vi "main(Test DQMH modules).bak.vi"() -> ()   [LabVIEW 2018, in "Application.lvlib"] (continued)
        n2853 = To Variant(anything=bool[] [FALSE, FALSE, FALSE, FALSE, FALSE, TRUE]) -> (Variant=w6353:variant)
        n2854 = To Variant(anything=T6."demux1_10_channel2" ("demux1_10(x6)_encode")) -> (Variant=w6357:variant)
        n2855 = To Variant(anything=T4."mux6_1_channel6_3" ("mux6_1(3wires)_encode")) -> (Variant=w6361:variant)
        n2856 = To Variant(anything=T5."mux10_1_channel2" ("mux10_1(x6)_encode")) -> (Variant=w6363:variant)
        n2857 = Bundle By Name(cluster=w6356, "command"="MEAS.mux10-1", "command data"=w6363) -> (w6351:T11)
        n2858 = Bundle By Name(cluster=w6356, "command"="MEAS.mux6_1", "command data"=w6361) -> (w6350:T11)
        n2859 = Bundle By Name(cluster=w6356, "command"="MEAS.demux1-10", "command data"=w6357) -> (w6349:T11)
        n2860 = Bundle By Name(cluster=w6356, "command"="MEAS.eMIC", "command data"=w6353) -> (w6348:T11)
        n2861 = Bundle By Name(cluster=w6356, "command"="MEAS.AllRelaysOFF") -> (w6352:T11)
        n2862 = Build Array(w6352, w6351, w6350, w6349, w6348) -> (w6343:T11[])
        n2863 = Bundle By Name(cluster=w6330, "command"="MEAS.requestAC", "command data"=w6324) -> (w6344:T11)
        n2864 = Bundle By Name(cluster=w6330, "command"="Apps.WaitForEvent", "command data"=w6324) -> (w6329:T11)
        n2865 = Bundle By Name(cluster=w6330, "command"="MEAS.DMM dual read") -> (w6345:T11)
        n2866 = Bundle By Name(cluster=w6330, "command"="Apps.UI Update 1") -> (w6331:T11)
        n2867 = Build Array(w6345, w6344, w6329, w6331) -> (w6342:T11[])
        n2868 = Build Array (concatenate)(w6343, w6342) -> (w6341:T11[])
        n2869 = for {
          tunnel: w6341 -> [w6379] mode=indexing
          tunnel: w6336 -> [w6380]
          tunnel: [w6376] -> w6339 mode=indexing
          n2870 = Unbundle By Name(w6379) -> ("command"=w6378:string, "command data"=w6377:variant)
          n2871 = call "App enquece.vi"("command data"=w6377, "command"=w6378, "queue in"=w6380) -> ("error out"=w6376:errorcluster)  [unwired: 7 in, 1 out]
        }
        n2872 = Merge Errors(w6340, w6339) -> (w6338:errorcluster)
      }
      frame "Test DRV 13A" {
        w6387 = T11 {"command"="", "command data"=variant} ("element")
        w6382 = 13 ("DUT index(0-59)")
        w6413 = T11 {"command"="", "command data"=variant} ("element")
        n2873 = disable-structure shown="LOGGING==TRUE" {
          disable-tunnel: w6391 -> [w6429 _]
          frame condition #0 (active) {
            n2874 = Empty String/Path?(string/path=w6429) -> (empty?=w6432:bool)
            n2875 = Select(t="Quece timeout", s=w6432, f=w6429) -> (s? t:f=w6428:string)
            n2876 = call "string log (SubVI).vi"("Enum"=enum16{"Init", "Log", "Read"}."Log", "state Name"=w6428) -> ()  [unwired: 8 in, 2 out]
          }
          frame condition #1 {
          }
        }
        n2877 = Flush Queue(queue=w6392) -> (queue out=w6393:refnum<queue>)  [unwired: 1 in, 2 out]
        n2878 = Decrement(x=w6382) -> (x-1=w6385:i32)
        n2879 = Index Array(array=w6381, index=w6385) -> (element=w6383:refnum<vi>)
        n2880 = property class="ColBox"(reference=w6383, "Value"=u32 10000536 ("DRV 1")) -> ()  [unwired: 1 in, 2 out]
        n2881 = To Variant(anything=bool[] [TRUE, FALSE, FALSE, FALSE, FALSE, FALSE]) -> (Variant=w6410:variant)
        n2882 = To Variant(anything=T6."demux1_10_channel3" ("demux1_10(x6)_encode")) -> (Variant=w6414:variant)
        n2883 = To Variant(anything=T4."mux6_1_channel1_3" ("mux6_1(3wires)_encode")) -> (Variant=w6418:variant)
        n2884 = To Variant(anything=T5."mux10_1_channel3" ("mux10_1(x6)_encode")) -> (Variant=w6420:variant)
        n2885 = Bundle By Name(cluster=w6413, "command"="MEAS.mux10-1", "command data"=w6420) -> (w6408:T11)
        n2886 = Bundle By Name(cluster=w6413, "command"="MEAS.mux6_1", "command data"=w6418) -> (w6407:T11)
        n2887 = Bundle By Name(cluster=w6413, "command"="MEAS.demux1-10", "command data"=w6414) -> (w6406:T11)
        n2888 = Bundle By Name(cluster=w6413, "command"="MEAS.eMIC", "command data"=w6410) -> (w6405:T11)
        n2889 = Bundle By Name(cluster=w6413, "command"="MEAS.AllRelaysOFF") -> (w6409:T11)
        n2890 = Build Array(w6409, w6408, w6407, w6406, w6405) -> (w6400:T11[])
        n2891 = Bundle By Name(cluster=w6387, "command"="MEAS.requestAC", "command data"=w6382) -> (w6401:T11)
        n2892 = Bundle By Name(cluster=w6387, "command"="Apps.WaitForEvent", "command data"=w6382) -> (w6386:T11)
        n2893 = Bundle By Name(cluster=w6387, "command"="MEAS.DMM dual read") -> (w6402:T11)
        n2894 = Bundle By Name(cluster=w6387, "command"="Apps.UI Update 1") -> (w6388:T11)
        n2895 = Build Array(w6402, w6401, w6386, w6388) -> (w6399:T11[])
        n2896 = Build Array (concatenate)(w6400, w6399) -> (w6398:T11[])
        n2897 = for {
          tunnel: w6398 -> [w6436] mode=indexing
          tunnel: w6393 -> [w6437]
          tunnel: [w6433] -> w6396 mode=indexing
          n2898 = Unbundle By Name(w6436) -> ("command"=w6435:string, "command data"=w6434:variant)
          n2899 = call "App enquece.vi"("command data"=w6434, "command"=w6435, "queue in"=w6437) -> ("error out"=w6433:errorcluster)  [unwired: 7 in, 1 out]
        }
        n2900 = Merge Errors(w6397, w6396) -> (w6395:errorcluster)
      }
      frame "Test DRV 14A" {
        w6444 = T11 {"command"="", "command data"=variant} ("element")
        w6439 = 14 ("DUT index(0-59)")
        w6470 = T11 {"command"="", "command data"=variant} ("element")
        n2901 = disable-structure shown="LOGGING==TRUE" {
          disable-tunnel: w6448 -> [w6486 _]
          frame condition #0 (active) {
            n2902 = Empty String/Path?(string/path=w6486) -> (empty?=w6489:bool)
            n2903 = Select(t="Quece timeout", s=w6489, f=w6486) -> (s? t:f=w6485:string)
            n2904 = call "string log (SubVI).vi"("Enum"=enum16{"Init", "Log", "Read"}."Log", "state Name"=w6485) -> ()  [unwired: 8 in, 2 out]
          }
          frame condition #1 {
          }
        }
        n2905 = Flush Queue(queue=w6449) -> (queue out=w6450:refnum<queue>)  [unwired: 1 in, 2 out]
        n2906 = Decrement(x=w6439) -> (x-1=w6442:i32)
        n2907 = Index Array(array=w6438, index=w6442) -> (element=w6440:refnum<vi>)
        n2908 = property class="ColBox"(reference=w6440, "Value"=u32 10000536 ("DRV 1")) -> ()  [unwired: 1 in, 2 out]
        n2909 = To Variant(anything=bool[] [FALSE, TRUE, FALSE, FALSE, FALSE, FALSE]) -> (Variant=w6467:variant)
        n2910 = To Variant(anything=T6."demux1_10_channel3" ("demux1_10(x6)_encode")) -> (Variant=w6471:variant)
        n2911 = To Variant(anything=T4."mux6_1_channel2_3" ("mux6_1(3wires)_encode")) -> (Variant=w6475:variant)
        n2912 = To Variant(anything=T5."mux10_1_channel3" ("mux10_1(x6)_encode")) -> (Variant=w6477:variant)
        n2913 = Bundle By Name(cluster=w6470, "command"="MEAS.mux10-1", "command data"=w6477) -> (w6465:T11)
        n2914 = Bundle By Name(cluster=w6470, "command"="MEAS.mux6_1", "command data"=w6475) -> (w6464:T11)
        n2915 = Bundle By Name(cluster=w6470, "command"="MEAS.demux1-10", "command data"=w6471) -> (w6463:T11)
        n2916 = Bundle By Name(cluster=w6470, "command"="MEAS.eMIC", "command data"=w6467) -> (w6462:T11)
        n2917 = Bundle By Name(cluster=w6470, "command"="MEAS.AllRelaysOFF") -> (w6466:T11)
        n2918 = Build Array(w6466, w6465, w6464, w6463, w6462) -> (w6457:T11[])
        n2919 = Bundle By Name(cluster=w6444, "command"="MEAS.requestAC", "command data"=w6439) -> (w6458:T11)
        n2920 = Bundle By Name(cluster=w6444, "command"="Apps.WaitForEvent", "command data"=w6439) -> (w6443:T11)
        n2921 = Bundle By Name(cluster=w6444, "command"="MEAS.DMM dual read") -> (w6459:T11)
        n2922 = Bundle By Name(cluster=w6444, "command"="Apps.UI Update 1") -> (w6445:T11)
        n2923 = Build Array(w6459, w6458, w6443, w6445) -> (w6456:T11[])
        n2924 = Build Array (concatenate)(w6457, w6456) -> (w6455:T11[])
        n2925 = for {
          tunnel: w6455 -> [w6493] mode=indexing
          tunnel: w6450 -> [w6494]
          tunnel: [w6490] -> w6453 mode=indexing
          n2926 = Unbundle By Name(w6493) -> ("command"=w6492:string, "command data"=w6491:variant)
          n2927 = call "App enquece.vi"("command data"=w6491, "command"=w6492, "queue in"=w6494) -> ("error out"=w6490:errorcluster)  [unwired: 7 in, 1 out]
        }
        n2928 = Merge Errors(w6454, w6453) -> (w6452:errorcluster)
      }
      frame "Test DRV 15A" {
        w6502 = T11 {"command"="", "command data"=variant} ("element")
        w6496 = 15 ("DUT index(0-59)")
        w6528 = T11 {"command"="", "command data"=variant} ("element")
        n2929 = disable-structure shown="LOGGING==TRUE" {
          disable-tunnel: w6506 -> [w6543 _]
          frame condition #0 (active) {
            n2930 = Empty String/Path?(string/path=w6543) -> (empty?=w6546:bool)
            n2931 = Select(t="Quece timeout", s=w6546, f=w6543) -> (s? t:f=w6542:string)
            n2932 = call "string log (SubVI).vi"("Enum"=enum16{"Init", "Log", "Read"}."Log", "state Name"=w6542) -> ()  [unwired: 8 in, 2 out]
          }
          frame condition #1 {
          }
        }
        n2933 = Flush Queue(queue=w6507) -> (queue out=w6508:refnum<queue>)  [unwired: 1 in, 2 out]
        n2934 = Decrement(x=w6496) -> (x-1=w6499:i32)
        n2935 = Index Array(array=w6495, index=w6499) -> (element=w6497:refnum<vi>)
        n2936 = property class="ColBox"(reference=w6497, "Value"=u32 10000536 ("DRV 1")) -> ()  [unwired: 1 in, 2 out]
        n2937 = To Variant(anything=bool[] [FALSE, FALSE, TRUE, FALSE, FALSE, FALSE]) -> (Variant=w6525:variant)
        n2938 = To Variant(anything=T6."demux1_10_channel3" ("demux1_10(x6)_encode")) -> (Variant=w6529:variant)
        n2939 = To Variant(anything=T4."mux6_1_channel3_3" ("mux6_1(3wires)_encode")) -> (Variant=w6532:variant)
        n2940 = To Variant(anything=T5."mux10_1_channel3" ("mux10_1(x6)_encode")) -> (Variant=w6534:variant)
        n2941 = Bundle By Name(cluster=w6528, "command"="MEAS.mux10-1", "command data"=w6534) -> (w6523:T11)
        n2942 = Bundle By Name(cluster=w6528, "command"="MEAS.mux6_1", "command data"=w6532) -> (w6522:T11)
        n2943 = Bundle By Name(cluster=w6528, "command"="MEAS.demux1-10", "command data"=w6529) -> (w6521:T11)
        n2944 = Bundle By Name(cluster=w6528, "command"="MEAS.eMIC", "command data"=w6525) -> (w6520:T11)
        n2945 = Bundle By Name(cluster=w6528, "command"="MEAS.AllRelaysOFF") -> (w6524:T11)
        n2946 = Build Array(w6524, w6523, w6522, w6521, w6520) -> (w6515:T11[])
        n2947 = Bundle By Name(cluster=w6502, "command"="MEAS.requestAC", "command data"=w6496) -> (w6516:T11)
        n2948 = Bundle By Name(cluster=w6502, "command"="Apps.WaitForEvent", "command data"=w6496) -> (w6501:T11)
        n2949 = Bundle By Name(cluster=w6502, "command"="MEAS.DMM dual read") -> (w6517:T11)
        n2950 = Bundle By Name(cluster=w6502, "command"="Apps.UI Update 1") -> (w6503:T11)
        n2951 = Build Array(w6517, w6516, w6501, w6503) -> (w6514:T11[])
        n2952 = Build Array (concatenate)(w6515, w6514) -> (w6513:T11[])
        n2953 = for {
          tunnel: w6513 -> [w6550] mode=indexing
          tunnel: w6508 -> [w6551]
          tunnel: [w6547] -> w6511 mode=indexing
          n2954 = Unbundle By Name(w6550) -> ("command"=w6549:string, "command data"=w6548:variant)
          n2955 = call "App enquece.vi"("command data"=w6548, "command"=w6549, "queue in"=w6551) -> ("error out"=w6547:errorcluster)  [unwired: 7 in, 1 out]
        }
        n2956 = Merge Errors(w6512, w6511) -> (w6510:errorcluster)
      }
      frame "Test DRV 16A" {
        w6559 = T11 {"command"="", "command data"=variant} ("element")
        w6553 = 16 ("DUT index(0-59)")
        w6585 = T11 {"command"="", "command data"=variant} ("element")
        n2957 = disable-structure shown="LOGGING==TRUE" {
          disable-tunnel: w6563 -> [w6600 _]
          frame condition #0 (active) {
            n2958 = Empty String/Path?(string/path=w6600) -> (empty?=w6603:bool)
            n2959 = Select(t="Quece timeout", s=w6603, f=w6600) -> (s? t:f=w6599:string)
            n2960 = call "string log (SubVI).vi"("Enum"=enum16{"Init", "Log", "Read"}."Log", "state Name"=w6599) -> ()  [unwired: 8 in, 2 out]
          }
          frame condition #1 {
          }
        }
        n2961 = Flush Queue(queue=w6564) -> (queue out=w6565:refnum<queue>)  [unwired: 1 in, 2 out]
        n2962 = Decrement(x=w6553) -> (x-1=w6556:i32)
        n2963 = Index Array(array=w6552, index=w6556) -> (element=w6554:refnum<vi>)
        n2964 = property class="ColBox"(reference=w6554, "Value"=u32 10000536 ("DRV 1")) -> ()  [unwired: 1 in, 2 out]
        n2965 = To Variant(anything=bool[] [FALSE, FALSE, FALSE, TRUE, FALSE, FALSE]) -> (Variant=w6582:variant)
        n2966 = To Variant(anything=T6."demux1_10_channel3" ("demux1_10(x6)_encode")) -> (Variant=w6586:variant)
        n2967 = To Variant(anything=T4."mux6_1_channel4_3" ("mux6_1(3wires)_encode")) -> (Variant=w6589:variant)
        n2968 = To Variant(anything=T5."mux10_1_channel3" ("mux10_1(x6)_encode")) -> (Variant=w6591:variant)
        n2969 = Bundle By Name(cluster=w6585, "command"="MEAS.mux10-1", "command data"=w6591) -> (w6580:T11)
        n2970 = Bundle By Name(cluster=w6585, "command"="MEAS.mux6_1", "command data"=w6589) -> (w6579:T11)
        n2971 = Bundle By Name(cluster=w6585, "command"="MEAS.demux1-10", "command data"=w6586) -> (w6578:T11)
        n2972 = Bundle By Name(cluster=w6585, "command"="MEAS.eMIC", "command data"=w6582) -> (w6577:T11)
        n2973 = Bundle By Name(cluster=w6585, "command"="MEAS.AllRelaysOFF") -> (w6581:T11)
        n2974 = Build Array(w6581, w6580, w6579, w6578, w6577) -> (w6572:T11[])
        n2975 = Bundle By Name(cluster=w6559, "command"="MEAS.requestAC", "command data"=w6553) -> (w6573:T11)
        n2976 = Bundle By Name(cluster=w6559, "command"="Apps.WaitForEvent", "command data"=w6553) -> (w6558:T11)
        n2977 = Bundle By Name(cluster=w6559, "command"="MEAS.DMM dual read") -> (w6574:T11)
        n2978 = Bundle By Name(cluster=w6559, "command"="Apps.UI Update 1") -> (w6560:T11)
        n2979 = Build Array(w6574, w6573, w6558, w6560) -> (w6571:T11[])
        n2980 = Build Array (concatenate)(w6572, w6571) -> (w6570:T11[])
        n2981 = for {
          tunnel: w6570 -> [w6607] mode=indexing
          tunnel: w6565 -> [w6608]
          tunnel: [w6604] -> w6568 mode=indexing
          n2982 = Unbundle By Name(w6607) -> ("command"=w6606:string, "command data"=w6605:variant)
          n2983 = call "App enquece.vi"("command data"=w6605, "command"=w6606, "queue in"=w6608) -> ("error out"=w6604:errorcluster)  [unwired: 7 in, 1 out]
        }
        n2984 = Merge Errors(w6569, w6568) -> (w6567:errorcluster)
      }
      frame "Test DRV 17A" {
        w6616 = T11 {"command"="", "command data"=variant} ("element")
        w6610 = 17 ("DUT index(0-59)")
        w6642 = T11 {"command"="", "command data"=variant} ("element")
        n2985 = disable-structure shown="LOGGING==TRUE" {
          disable-tunnel: w6620 -> [w6657 _]
          frame condition #0 (active) {
            n2986 = Empty String/Path?(string/path=w6657) -> (empty?=w6660:bool)
            n2987 = Select(t="Quece timeout", s=w6660, f=w6657) -> (s? t:f=w6656:string)
            n2988 = call "string log (SubVI).vi"("Enum"=enum16{"Init", "Log", "Read"}."Log", "state Name"=w6656) -> ()  [unwired: 8 in, 2 out]
          }
          frame condition #1 {
          }
        }
        n2989 = Flush Queue(queue=w6621) -> (queue out=w6622:refnum<queue>)  [unwired: 1 in, 2 out]
        n2990 = Decrement(x=w6610) -> (x-1=w6613:i32)
        n2991 = Index Array(array=w6609, index=w6613) -> (element=w6611:refnum<vi>)
        n2992 = property class="ColBox"(reference=w6611, "Value"=u32 10000536 ("DRV 1")) -> ()  [unwired: 1 in, 2 out]
        n2993 = To Variant(anything=bool[] [FALSE, FALSE, FALSE, FALSE, TRUE, FALSE]) -> (Variant=w6639:variant)
        n2994 = To Variant(anything=T6."demux1_10_channel3" ("demux1_10(x6)_encode")) -> (Variant=w6643:variant)
        n2995 = To Variant(anything=T4."mux6_1_channel5_3" ("mux6_1(3wires)_encode")) -> (Variant=w6646:variant)
        n2996 = To Variant(anything=T5."mux10_1_channel3" ("mux10_1(x6)_encode")) -> (Variant=w6648:variant)
        n2997 = Bundle By Name(cluster=w6642, "command"="MEAS.mux10-1", "command data"=w6648) -> (w6637:T11)
        n2998 = Bundle By Name(cluster=w6642, "command"="MEAS.mux6_1", "command data"=w6646) -> (w6636:T11)
        n2999 = Bundle By Name(cluster=w6642, "command"="MEAS.demux1-10", "command data"=w6643) -> (w6635:T11)
        n3000 = Bundle By Name(cluster=w6642, "command"="MEAS.eMIC", "command data"=w6639) -> (w6634:T11)
        n3001 = Bundle By Name(cluster=w6642, "command"="MEAS.AllRelaysOFF") -> (w6638:T11)
        n3002 = Build Array(w6638, w6637, w6636, w6635, w6634) -> (w6629:T11[])
        n3003 = Bundle By Name(cluster=w6616, "command"="Apps.WaitForEvent", "command data"=w6610) -> (w6615:T11)
        n3004 = Bundle By Name(cluster=w6616, "command"="MEAS.requestAC", "command data"=w6610) -> (w6630:T11)
        n3005 = Bundle By Name(cluster=w6616, "command"="Apps.UI Update 1") -> (w6617:T11)
        n3006 = Bundle By Name(cluster=w6616, "command"="MEAS.DMM dual read") -> (w6631:T11)
        n3007 = Build Array(w6631, w6630, w6615, w6617) -> (w6628:T11[])
        n3008 = Build Array (concatenate)(w6629, w6628) -> (w6627:T11[])
        n3009 = for {
          tunnel: w6627 -> [w6664] mode=indexing
          tunnel: w6622 -> [w6665]
          tunnel: [w6661] -> w6625 mode=indexing
          n3010 = Unbundle By Name(w6664) -> ("command"=w6663:string, "command data"=w6662:variant)
          n3011 = call "App enquece.vi"("command data"=w6662, "command"=w6663, "queue in"=w6665) -> ("error out"=w6661:errorcluster)  [unwired: 7 in, 1 out]
        }
        n3012 = Merge Errors(w6626, w6625) -> (w6624:errorcluster)
      }
      frame "Test DRV 18A" {
        w6673 = T11 {"command"="", "command data"=variant} ("element")
        w6667 = 18 ("DUT index(0-59)")
        w6699 = T11 {"command"="", "command data"=variant} ("element")
        n3013 = disable-structure shown="LOGGING==TRUE" {
          disable-tunnel: w6677 -> [w6714 _]
          frame condition #0 (active) {
            n3014 = Empty String/Path?(string/path=w6714) -> (empty?=w6717:bool)
            n3015 = Select(t="Quece timeout", s=w6717, f=w6714) -> (s? t:f=w6713:string)
            n3016 = call "string log (SubVI).vi"("Enum"=enum16{"Init", "Log", "Read"}."Log", "state Name"=w6713) -> ()  [unwired: 8 in, 2 out]
          }
          frame condition #1 {
          }
        }
        n3017 = Flush Queue(queue=w6678) -> (queue out=w6679:refnum<queue>)  [unwired: 1 in, 2 out]
        n3018 = Decrement(x=w6667) -> (x-1=w6670:i32)
        n3019 = Index Array(array=w6666, index=w6670) -> (element=w6668:refnum<vi>)
        n3020 = property class="ColBox"(reference=w6668, "Value"=u32 10000536 ("DRV 1")) -> ()  [unwired: 1 in, 2 out]
        n3021 = To Variant(anything=bool[] [FALSE, FALSE, FALSE, FALSE, FALSE, TRUE]) -> (Variant=w6696:variant)
        n3022 = To Variant(anything=T6."demux1_10_channel3" ("demux1_10(x6)_encode")) -> (Variant=w6700:variant)
        n3023 = To Variant(anything=T4."mux6_1_channel6_3" ("mux6_1(3wires)_encode")) -> (Variant=w6703:variant)
        n3024 = To Variant(anything=T5."mux10_1_channel3" ("mux10_1(x6)_encode")) -> (Variant=w6705:variant)
        n3025 = Bundle By Name(cluster=w6699, "command"="MEAS.mux10-1", "command data"=w6705) -> (w6694:T11)
        n3026 = Bundle By Name(cluster=w6699, "command"="MEAS.mux6_1", "command data"=w6703) -> (w6693:T11)
        n3027 = Bundle By Name(cluster=w6699, "command"="MEAS.demux1-10", "command data"=w6700) -> (w6692:T11)
        n3028 = Bundle By Name(cluster=w6699, "command"="MEAS.eMIC", "command data"=w6696) -> (w6691:T11)
        n3029 = Bundle By Name(cluster=w6699, "command"="MEAS.AllRelaysOFF") -> (w6695:T11)
        n3030 = Build Array(w6695, w6694, w6693, w6692, w6691) -> (w6686:T11[])
        n3031 = Bundle By Name(cluster=w6673, "command"="MEAS.requestAC", "command data"=w6667) -> (w6687:T11)
        n3032 = Bundle By Name(cluster=w6673, "command"="Apps.WaitForEvent", "command data"=w6667) -> (w6672:T11)
        n3033 = Bundle By Name(cluster=w6673, "command"="MEAS.DMM dual read") -> (w6688:T11)
        n3034 = Bundle By Name(cluster=w6673, "command"="Apps.UI Update 1") -> (w6674:T11)
        n3035 = Build Array(w6688, w6687, w6672, w6674) -> (w6685:T11[])
        n3036 = Build Array (concatenate)(w6686, w6685) -> (w6684:T11[])
        n3037 = for {
          tunnel: w6684 -> [w6721] mode=indexing
          tunnel: w6679 -> [w6722]
          tunnel: [w6718] -> w6682 mode=indexing
          n3038 = Unbundle By Name(w6721) -> ("command"=w6720:string, "command data"=w6719:variant)
          n3039 = call "App enquece.vi"("command data"=w6719, "command"=w6720, "queue in"=w6722) -> ("error out"=w6718:errorcluster)  [unwired: 7 in, 1 out]
        }
        n3040 = Merge Errors(w6683, w6682) -> (w6681:errorcluster)
      }
      frame "Test DRV 19A" {
        w6730 = T11 {"command"="", "command data"=variant} ("element")
        w6724 = 19 ("DUT index(0-59)")
        w6756 = T11 {"command"="", "command data"=variant} ("element")
        n3041 = disable-structure shown="LOGGING==TRUE" {
          disable-tunnel: w6734 -> [w6771 _]
          frame condition #0 (active) {
            n3042 = Empty String/Path?(string/path=w6771) -> (empty?=w6774:bool)
            n3043 = Select(t="Quece timeout", s=w6774, f=w6771) -> (s? t:f=w6770:string)
            n3044 = call "string log (SubVI).vi"("Enum"=enum16{"Init", "Log", "Read"}."Log", "state Name"=w6770) -> ()  [unwired: 8 in, 2 out]
          }
          frame condition #1 {
          }
        }
        n3045 = Flush Queue(queue=w6735) -> (queue out=w6736:refnum<queue>)  [unwired: 1 in, 2 out]
        n3046 = Decrement(x=w6724) -> (x-1=w6727:i32)
        n3047 = Index Array(array=w6723, index=w6727) -> (element=w6725:refnum<vi>)
        n3048 = property class="ColBox"(reference=w6725, "Value"=u32 10000536 ("DRV 1")) -> ()  [unwired: 1 in, 2 out]
        n3049 = To Variant(anything=bool[] [TRUE, FALSE, FALSE, FALSE, FALSE, FALSE]) -> (Variant=w6753:variant)
        n3050 = To Variant(anything=T6."demux1_10_channel4" ("demux1_10(x6)_encode")) -> (Variant=w6757:variant)
        n3051 = To Variant(anything=T4."mux6_1_channel1_3" ("mux6_1(3wires)_encode")) -> (Variant=w6760:variant)
        n3052 = To Variant(anything=T5."mux10_1_channel4" ("mux10_1(x6)_encode")) -> (Variant=w6762:variant)
        n3053 = Bundle By Name(cluster=w6756, "command"="MEAS.mux10-1", "command data"=w6762) -> (w6751:T11)
        n3054 = Bundle By Name(cluster=w6756, "command"="MEAS.mux6_1", "command data"=w6760) -> (w6750:T11)
        n3055 = Bundle By Name(cluster=w6756, "command"="MEAS.demux1-10", "command data"=w6757) -> (w6749:T11)
        n3056 = Bundle By Name(cluster=w6756, "command"="MEAS.eMIC", "command data"=w6753) -> (w6748:T11)
        n3057 = Bundle By Name(cluster=w6756, "command"="MEAS.AllRelaysOFF") -> (w6752:T11)
        n3058 = Build Array(w6752, w6751, w6750, w6749, w6748) -> (w6743:T11[])
        n3059 = Bundle By Name(cluster=w6730, "command"="MEAS.requestAC", "command data"=w6724) -> (w6744:T11)
        n3060 = Bundle By Name(cluster=w6730, "command"="Apps.WaitForEvent", "command data"=w6724) -> (w6729:T11)
        n3061 = Bundle By Name(cluster=w6730, "command"="MEAS.DMM dual read") -> (w6745:T11)
        n3062 = Bundle By Name(cluster=w6730, "command"="Apps.UI Update 1") -> (w6731:T11)
        n3063 = Build Array(w6745, w6744, w6729, w6731) -> (w6742:T11[])
        n3064 = Build Array (concatenate)(w6743, w6742) -> (w6741:T11[])
        n3065 = for {
          tunnel: w6741 -> [w6778] mode=indexing
          tunnel: w6736 -> [w6779]
          tunnel: [w6775] -> w6739 mode=indexing
          n3066 = Unbundle By Name(w6778) -> ("command"=w6777:string, "command data"=w6776:variant)
          n3067 = call "App enquece.vi"("command data"=w6776, "command"=w6777, "queue in"=w6779) -> ("error out"=w6775:errorcluster)  [unwired: 7 in, 1 out]
        }
        n3068 = Merge Errors(w6740, w6739) -> (w6738:errorcluster)
      }
      frame "Test DRV 20A" {
        w6787 = T11 {"command"="", "command data"=variant} ("element")
        w6781 = 20 ("DUT index(0-59)")
        w6813 = T11 {"command"="", "command data"=variant} ("element")
        n3069 = disable-structure shown="LOGGING==TRUE" {
          disable-tunnel: w6791 -> [w6828 _]
          frame condition #0 (active) {
            n3070 = Empty String/Path?(string/path=w6828) -> (empty?=w6831:bool)
            n3071 = Select(t="Quece timeout", s=w6831, f=w6828) -> (s? t:f=w6827:string)
            n3072 = call "string log (SubVI).vi"("Enum"=enum16{"Init", "Log", "Read"}."Log", "state Name"=w6827) -> ()  [unwired: 8 in, 2 out]
          }
          frame condition #1 {
          }
        }
        n3073 = Flush Queue(queue=w6792) -> (queue out=w6793:refnum<queue>)  [unwired: 1 in, 2 out]
        n3074 = Decrement(x=w6781) -> (x-1=w6784:i32)
        n3075 = Index Array(array=w6780, index=w6784) -> (element=w6782:refnum<vi>)
        n3076 = property class="ColBox"(reference=w6782, "Value"=u32 10000536 ("DRV 1")) -> ()  [unwired: 1 in, 2 out]
        n3077 = To Variant(anything=bool[] [FALSE, TRUE, FALSE, FALSE, FALSE, FALSE]) -> (Variant=w6810:variant)
        n3078 = To Variant(anything=T6."demux1_10_channel4" ("demux1_10(x6)_encode")) -> (Variant=w6814:variant)
        n3079 = To Variant(anything=T4."mux6_1_channel2_3" ("mux6_1(3wires)_encode")) -> (Variant=w6817:variant)
        n3080 = To Variant(anything=T5."mux10_1_channel4" ("mux10_1(x6)_encode")) -> (Variant=w6819:variant)
        n3081 = Bundle By Name(cluster=w6813, "command"="MEAS.mux10-1", "command data"=w6819) -> (w6808:T11)
        n3082 = Bundle By Name(cluster=w6813, "command"="MEAS.mux6_1", "command data"=w6817) -> (w6807:T11)
        n3083 = Bundle By Name(cluster=w6813, "command"="MEAS.demux1-10", "command data"=w6814) -> (w6806:T11)
        n3084 = Bundle By Name(cluster=w6813, "command"="MEAS.eMIC", "command data"=w6810) -> (w6805:T11)
        n3085 = Bundle By Name(cluster=w6813, "command"="MEAS.AllRelaysOFF") -> (w6809:T11)
        n3086 = Build Array(w6809, w6808, w6807, w6806, w6805) -> (w6800:T11[])
        n3087 = Bundle By Name(cluster=w6787, "command"="MEAS.requestAC", "command data"=w6781) -> (w6801:T11)
        n3088 = Bundle By Name(cluster=w6787, "command"="Apps.WaitForEvent", "command data"=w6781) -> (w6786:T11)
        n3089 = Bundle By Name(cluster=w6787, "command"="MEAS.DMM dual read") -> (w6802:T11)
        n3090 = Bundle By Name(cluster=w6787, "command"="Apps.UI Update 1") -> (w6788:T11)
        n3091 = Build Array(w6802, w6801, w6786, w6788) -> (w6799:T11[])
        n3092 = Build Array (concatenate)(w6800, w6799) -> (w6798:T11[])
        n3093 = for {
          tunnel: w6798 -> [w6835] mode=indexing
          tunnel: w6793 -> [w6836]
          tunnel: [w6832] -> w6796 mode=indexing
          n3094 = Unbundle By Name(w6835) -> ("command"=w6834:string, "command data"=w6833:variant)
          n3095 = call "App enquece.vi"("command data"=w6833, "command"=w6834, "queue in"=w6836) -> ("error out"=w6832:errorcluster)  [unwired: 7 in, 1 out]
        }
        n3096 = Merge Errors(w6797, w6796) -> (w6795:errorcluster)
      }
      frame "Test DRV 21A" {
        w6844 = T11 {"command"="", "command data"=variant} ("element")
        w6837 = 21 ("DUT index(0-59)")
        w6870 = T11 {"command"="", "command data"=variant} ("element")
        n3097 = disable-structure shown="LOGGING==TRUE" {
          disable-tunnel: w6848 -> [w6885 _]
          frame condition #0 (active) {
            n3098 = Empty String/Path?(string/path=w6885) -> (empty?=w6888:bool)
            n3099 = Select(t="Quece timeout", s=w6888, f=w6885) -> (s? t:f=w6884:string)
            n3100 = call "string log (SubVI).vi"("Enum"=enum16{"Init", "Log", "Read"}."Log", "state Name"=w6884) -> ()  [unwired: 8 in, 2 out]
          }
          frame condition #1 {
          }
        }
        n3101 = Flush Queue(queue=w6849) -> (queue out=w6850:refnum<queue>)  [unwired: 1 in, 2 out]
        n3102 = Decrement(x=w6837) -> (x-1=w6841:i32)
        n3103 = Index Array(array=w6838, index=w6841) -> (element=w6839:refnum<vi>)
        n3104 = property class="ColBox"(reference=w6839, "Value"=u32 10000536 ("DRV 1")) -> ()  [unwired: 1 in, 2 out]
        n3105 = To Variant(anything=bool[] [FALSE, FALSE, TRUE, FALSE, FALSE, FALSE]) -> (Variant=w6867:variant)
        n3106 = To Variant(anything=T6."demux1_10_channel4" ("demux1_10(x6)_encode")) -> (Variant=w6871:variant)
        n3107 = To Variant(anything=T4."mux6_1_channel3_3" ("mux6_1(3wires)_encode")) -> (Variant=w6874:variant)
        n3108 = To Variant(anything=T5."mux10_1_channel4" ("mux10_1(x6)_encode")) -> (Variant=w6876:variant)
        n3109 = Bundle By Name(cluster=w6870, "command"="MEAS.mux10-1", "command data"=w6876) -> (w6865:T11)
        n3110 = Bundle By Name(cluster=w6870, "command"="MEAS.mux6_1", "command data"=w6874) -> (w6864:T11)
        n3111 = Bundle By Name(cluster=w6870, "command"="MEAS.demux1-10", "command data"=w6871) -> (w6863:T11)
        n3112 = Bundle By Name(cluster=w6870, "command"="MEAS.eMIC", "command data"=w6867) -> (w6862:T11)
        n3113 = Bundle By Name(cluster=w6870, "command"="MEAS.AllRelaysOFF") -> (w6866:T11)
        n3114 = Build Array(w6866, w6865, w6864, w6863, w6862) -> (w6857:T11[])
        n3115 = Bundle By Name(cluster=w6844, "command"="MEAS.requestAC", "command data"=w6837) -> (w6858:T11)
        n3116 = Bundle By Name(cluster=w6844, "command"="Apps.WaitForEvent", "command data"=w6837) -> (w6843:T11)
        n3117 = Bundle By Name(cluster=w6844, "command"="MEAS.DMM dual read") -> (w6859:T11)
        n3118 = Bundle By Name(cluster=w6844, "command"="Apps.UI Update 1") -> (w6845:T11)
        n3119 = Build Array(w6859, w6858, w6843, w6845) -> (w6856:T11[])
        n3120 = Build Array (concatenate)(w6857, w6856) -> (w6855:T11[])
        n3121 = for {
          tunnel: w6855 -> [w6892] mode=indexing
          tunnel: w6850 -> [w6893]
          tunnel: [w6889] -> w6853 mode=indexing
          n3122 = Unbundle By Name(w6892) -> ("command"=w6891:string, "command data"=w6890:variant)
          n3123 = call "App enquece.vi"("command data"=w6890, "command"=w6891, "queue in"=w6893) -> ("error out"=w6889:errorcluster)  [unwired: 7 in, 1 out]
        }
        n3124 = Merge Errors(w6854, w6853) -> (w6852:errorcluster)
      }
      frame "Test DRV 22A" {
        w6901 = T11 {"command"="", "command data"=variant} ("element")
        w6895 = 22 ("DUT index(0-59)")
        w6927 = T11 {"command"="", "command data"=variant} ("element")
        n3125 = disable-structure shown="LOGGING==TRUE" {
          disable-tunnel: w6905 -> [w6942 _]
          frame condition #0 (active) {
            n3126 = Empty String/Path?(string/path=w6942) -> (empty?=w6945:bool)
            n3127 = Select(t="Quece timeout", s=w6945, f=w6942) -> (s? t:f=w6941:string)
            n3128 = call "string log (SubVI).vi"("Enum"=enum16{"Init", "Log", "Read"}."Log", "state Name"=w6941) -> ()  [unwired: 8 in, 2 out]
          }
          frame condition #1 {
          }
        }
        n3129 = Flush Queue(queue=w6906) -> (queue out=w6907:refnum<queue>)  [unwired: 1 in, 2 out]
        n3130 = Decrement(x=w6895) -> (x-1=w6898:i32)
        n3131 = Index Array(array=w6894, index=w6898) -> (element=w6896:refnum<vi>)
        n3132 = property class="ColBox"(reference=w6896, "Value"=u32 10000536 ("DRV 1")) -> ()  [unwired: 1 in, 2 out]
        n3133 = To Variant(anything=bool[] [FALSE, FALSE, FALSE, TRUE, FALSE, FALSE]) -> (Variant=w6924:variant)
        n3134 = To Variant(anything=T6."demux1_10_channel4" ("demux1_10(x6)_encode")) -> (Variant=w6928:variant)
        n3135 = To Variant(anything=T4."mux6_1_channel4_3" ("mux6_1(3wires)_encode")) -> (Variant=w6931:variant)
        n3136 = To Variant(anything=T5."mux10_1_channel4" ("mux10_1(x6)_encode")) -> (Variant=w6933:variant)
        n3137 = Bundle By Name(cluster=w6927, "command"="MEAS.mux10-1", "command data"=w6933) -> (w6922:T11)
        n3138 = Bundle By Name(cluster=w6927, "command"="MEAS.mux6_1", "command data"=w6931) -> (w6921:T11)
        n3139 = Bundle By Name(cluster=w6927, "command"="MEAS.demux1-10", "command data"=w6928) -> (w6920:T11)
        n3140 = Bundle By Name(cluster=w6927, "command"="MEAS.eMIC", "command data"=w6924) -> (w6919:T11)
        n3141 = Bundle By Name(cluster=w6927, "command"="MEAS.AllRelaysOFF") -> (w6923:T11)
        n3142 = Build Array(w6923, w6922, w6921, w6920, w6919) -> (w6914:T11[])
        n3143 = Bundle By Name(cluster=w6901, "command"="MEAS.requestAC", "command data"=w6895) -> (w6915:T11)
        n3144 = Bundle By Name(cluster=w6901, "command"="Apps.WaitForEvent", "command data"=w6895) -> (w6900:T11)
        n3145 = Bundle By Name(cluster=w6901, "command"="MEAS.DMM dual read") -> (w6916:T11)
        n3146 = Bundle By Name(cluster=w6901, "command"="Apps.UI Update 1") -> (w6902:T11)
        n3147 = Build Array(w6916, w6915, w6900, w6902) -> (w6913:T11[])
        n3148 = Build Array (concatenate)(w6914, w6913) -> (w6912:T11[])
        n3149 = for {
          tunnel: w6912 -> [w6949] mode=indexing
          tunnel: w6907 -> [w6950]
          tunnel: [w6946] -> w6910 mode=indexing
          n3150 = Unbundle By Name(w6949) -> ("command"=w6948:string, "command data"=w6947:variant)
          n3151 = call "App enquece.vi"("command data"=w6947, "command"=w6948, "queue in"=w6950) -> ("error out"=w6946:errorcluster)  [unwired: 7 in, 1 out]
        }
        n3152 = Merge Errors(w6911, w6910) -> (w6909:errorcluster)
      }
      frame "Test DRV 23A" {
        w6958 = T11 {"command"="", "command data"=variant} ("element")
        w6951 = 23 ("DUT index(0-59)")
        w6984 = T11 {"command"="", "command data"=variant} ("element")
        n3153 = disable-structure shown="LOGGING==TRUE" {
          disable-tunnel: w6962 -> [w6999 _]
          frame condition #0 (active) {
            n3154 = Empty String/Path?(string/path=w6999) -> (empty?=w7002:bool)
            n3155 = Select(t="Quece timeout", s=w7002, f=w6999) -> (s? t:f=w6998:string)
            n3156 = call "string log (SubVI).vi"("Enum"=enum16{"Init", "Log", "Read"}."Log", "state Name"=w6998) -> ()  [unwired: 8 in, 2 out]
          }
          frame condition #1 {
          }
        }
        n3157 = Flush Queue(queue=w6963) -> (queue out=w6964:refnum<queue>)  [unwired: 1 in, 2 out]
        n3158 = Decrement(x=w6951) -> (x-1=w6955:i32)
        n3159 = Index Array(array=w6952, index=w6955) -> (element=w6953:refnum<vi>)
        n3160 = property class="ColBox"(reference=w6953, "Value"=u32 10000536 ("DRV 1")) -> ()  [unwired: 1 in, 2 out]
        n3161 = To Variant(anything=bool[] [FALSE, FALSE, FALSE, FALSE, TRUE, FALSE]) -> (Variant=w6981:variant)
        n3162 = To Variant(anything=T6."demux1_10_channel4" ("demux1_10(x6)_encode")) -> (Variant=w6985:variant)
        n3163 = To Variant(anything=T4."mux6_1_channel5_3" ("mux6_1(3wires)_encode")) -> (Variant=w6988:variant)
        n3164 = To Variant(anything=T5."mux10_1_channel4" ("mux10_1(x6)_encode")) -> (Variant=w6990:variant)
        n3165 = Bundle By Name(cluster=w6984, "command"="MEAS.mux10-1", "command data"=w6990) -> (w6979:T11)
        n3166 = Bundle By Name(cluster=w6984, "command"="MEAS.mux6_1", "command data"=w6988) -> (w6978:T11)
        n3167 = Bundle By Name(cluster=w6984, "command"="MEAS.demux1-10", "command data"=w6985) -> (w6977:T11)
        n3168 = Bundle By Name(cluster=w6984, "command"="MEAS.eMIC", "command data"=w6981) -> (w6976:T11)
        n3169 = Bundle By Name(cluster=w6984, "command"="MEAS.AllRelaysOFF") -> (w6980:T11)
        n3170 = Build Array(w6980, w6979, w6978, w6977, w6976) -> (w6971:T11[])
        n3171 = Bundle By Name(cluster=w6958, "command"="MEAS.requestAC", "command data"=w6951) -> (w6972:T11)
        n3172 = Bundle By Name(cluster=w6958, "command"="Apps.WaitForEvent", "command data"=w6951) -> (w6957:T11)
        n3173 = Bundle By Name(cluster=w6958, "command"="MEAS.DMM dual read") -> (w6973:T11)
        n3174 = Bundle By Name(cluster=w6958, "command"="Apps.UI Update 1") -> (w6959:T11)
        n3175 = Build Array(w6973, w6972, w6957, w6959) -> (w6970:T11[])
        n3176 = Build Array (concatenate)(w6971, w6970) -> (w6969:T11[])
        n3177 = for {
          tunnel: w6969 -> [w7006] mode=indexing
          tunnel: w6964 -> [w7007]
          tunnel: [w7003] -> w6967 mode=indexing
          n3178 = Unbundle By Name(w7006) -> ("command"=w7005:string, "command data"=w7004:variant)
          n3179 = call "App enquece.vi"("command data"=w7004, "command"=w7005, "queue in"=w7007) -> ("error out"=w7003:errorcluster)  [unwired: 7 in, 1 out]
        }
        n3180 = Merge Errors(w6968, w6967) -> (w6966:errorcluster)
      }
      frame "Test DRV 24A" {
        w7015 = T11 {"command"="", "command data"=variant} ("element")
        w7008 = 24 ("DUT index(0-59)")
        w7041 = T11 {"command"="", "command data"=variant} ("element")
        n3181 = disable-structure shown="LOGGING==TRUE" {
          disable-tunnel: w7019 -> [w7056 _]
          frame condition #0 (active) {
            n3182 = Empty String/Path?(string/path=w7056) -> (empty?=w7059:bool)
            n3183 = Select(t="Quece timeout", s=w7059, f=w7056) -> (s? t:f=w7055:string)
            n3184 = call "string log (SubVI).vi"("Enum"=enum16{"Init", "Log", "Read"}."Log", "state Name"=w7055) -> ()  [unwired: 8 in, 2 out]
          }
          frame condition #1 {
          }
        }
        n3185 = Flush Queue(queue=w7020) -> (queue out=w7021:refnum<queue>)  [unwired: 1 in, 2 out]
        n3186 = Decrement(x=w7008) -> (x-1=w7012:i32)
        n3187 = Index Array(array=w7009, index=w7012) -> (element=w7010:refnum<vi>)
        n3188 = property class="ColBox"(reference=w7010, "Value"=u32 10000536 ("DRV 1")) -> ()  [unwired: 1 in, 2 out]
        n3189 = To Variant(anything=bool[] [FALSE, FALSE, FALSE, FALSE, FALSE, TRUE]) -> (Variant=w7038:variant)
        n3190 = To Variant(anything=T6."demux1_10_channel4" ("demux1_10(x6)_encode")) -> (Variant=w7042:variant)
        n3191 = To Variant(anything=T4."mux6_1_channel6_3" ("mux6_1(3wires)_encode")) -> (Variant=w7045:variant)
        n3192 = To Variant(anything=T5."mux10_1_channel4" ("mux10_1(x6)_encode")) -> (Variant=w7047:variant)
        n3193 = Bundle By Name(cluster=w7041, "command"="MEAS.mux10-1", "command data"=w7047) -> (w7036:T11)
        n3194 = Bundle By Name(cluster=w7041, "command"="MEAS.mux6_1", "command data"=w7045) -> (w7035:T11)
        n3195 = Bundle By Name(cluster=w7041, "command"="MEAS.demux1-10", "command data"=w7042) -> (w7034:T11)
        n3196 = Bundle By Name(cluster=w7041, "command"="MEAS.eMIC", "command data"=w7038) -> (w7033:T11)
        n3197 = Bundle By Name(cluster=w7041, "command"="MEAS.AllRelaysOFF") -> (w7037:T11)
        n3198 = Build Array(w7037, w7036, w7035, w7034, w7033) -> (w7028:T11[])
        n3199 = Bundle By Name(cluster=w7015, "command"="MEAS.requestAC", "command data"=w7008) -> (w7029:T11)
        n3200 = Bundle By Name(cluster=w7015, "command"="Apps.WaitForEvent", "command data"=w7008) -> (w7014:T11)
        n3201 = Bundle By Name(cluster=w7015, "command"="MEAS.DMM dual read") -> (w7030:T11)
        n3202 = Bundle By Name(cluster=w7015, "command"="Apps.UI Update 1") -> (w7016:T11)
        n3203 = Build Array(w7030, w7029, w7014, w7016) -> (w7027:T11[])
        n3204 = Build Array (concatenate)(w7028, w7027) -> (w7026:T11[])
        n3205 = for {
          tunnel: w7026 -> [w7063] mode=indexing
          tunnel: w7021 -> [w7064]
          tunnel: [w7060] -> w7024 mode=indexing
          n3206 = Unbundle By Name(w7063) -> ("command"=w7062:string, "command data"=w7061:variant)
          n3207 = call "App enquece.vi"("command data"=w7061, "command"=w7062, "queue in"=w7064) -> ("error out"=w7060:errorcluster)  [unwired: 7 in, 1 out]
        }
        n3208 = Merge Errors(w7025, w7024) -> (w7023:errorcluster)
      }
      frame "Test DRV 25A" {
        w7072 = T11 {"command"="", "command data"=variant} ("element")
        w7066 = 25 ("DUT index(0-59)")
        w7098 = T11 {"command"="", "command data"=variant} ("element")
        n3209 = disable-structure shown="LOGGING==TRUE" {
          disable-tunnel: w7076 -> [w7113 _]
          frame condition #0 (active) {
            n3210 = Empty String/Path?(string/path=w7113) -> (empty?=w7116:bool)
            n3211 = Select(t="Quece timeout", s=w7116, f=w7113) -> (s? t:f=w7112:string)
            n3212 = call "string log (SubVI).vi"("Enum"=enum16{"Init", "Log", "Read"}."Log", "state Name"=w7112) -> ()  [unwired: 8 in, 2 out]
          }
          frame condition #1 {
          }
        }
        n3213 = Flush Queue(queue=w7077) -> (queue out=w7078:refnum<queue>)  [unwired: 1 in, 2 out]
        n3214 = Decrement(x=w7066) -> (x-1=w7069:i32)
        n3215 = Index Array(array=w7065, index=w7069) -> (element=w7067:refnum<vi>)
        n3216 = property class="ColBox"(reference=w7067, "Value"=u32 10000536 ("DRV 1")) -> ()  [unwired: 1 in, 2 out]
        n3217 = To Variant(anything=bool[] [TRUE, FALSE, FALSE, FALSE, FALSE, FALSE]) -> (Variant=w7095:variant)
        n3218 = To Variant(anything=T6."demux1_10_channel5" ("demux1_10(x6)_encode")) -> (Variant=w7099:variant)
        n3219 = To Variant(anything=T4."mux6_1_channel1_3" ("mux6_1(3wires)_encode")) -> (Variant=w7102:variant)
        n3220 = To Variant(anything=T5."mux10_1_channel5" ("mux10_1(x6)_encode")) -> (Variant=w7104:variant)
        n3221 = Bundle By Name(cluster=w7098, "command"="MEAS.mux10-1", "command data"=w7104) -> (w7093:T11)
        n3222 = Bundle By Name(cluster=w7098, "command"="MEAS.mux6_1", "command data"=w7102) -> (w7092:T11)
        n3223 = Bundle By Name(cluster=w7098, "command"="MEAS.demux1-10", "command data"=w7099) -> (w7091:T11)
        n3224 = Bundle By Name(cluster=w7098, "command"="MEAS.eMIC", "command data"=w7095) -> (w7090:T11)
        n3225 = Bundle By Name(cluster=w7098, "command"="MEAS.AllRelaysOFF") -> (w7094:T11)
        n3226 = Build Array(w7094, w7093, w7092, w7091, w7090) -> (w7085:T11[])
        n3227 = Bundle By Name(cluster=w7072, "command"="MEAS.requestAC", "command data"=w7066) -> (w7086:T11)
        n3228 = Bundle By Name(cluster=w7072, "command"="Apps.WaitForEvent", "command data"=w7066) -> (w7071:T11)
        n3229 = Bundle By Name(cluster=w7072, "command"="MEAS.DMM dual read") -> (w7087:T11)
        n3230 = Bundle By Name(cluster=w7072, "command"="Apps.UI Update 1") -> (w7073:T11)
        n3231 = Build Array(w7087, w7086, w7071, w7073) -> (w7084:T11[])
        n3232 = Build Array (concatenate)(w7085, w7084) -> (w7083:T11[])
        n3233 = for {
          tunnel: w7083 -> [w7120] mode=indexing
          tunnel: w7078 -> [w7121]
          tunnel: [w7117] -> w7081 mode=indexing
          n3234 = Unbundle By Name(w7120) -> ("command"=w7119:string, "command data"=w7118:variant)
          n3235 = call "App enquece.vi"("command data"=w7118, "command"=w7119, "queue in"=w7121) -> ("error out"=w7117:errorcluster)  [unwired: 7 in, 1 out]
        }
        n3236 = Merge Errors(w7082, w7081) -> (w7080:errorcluster)
      }
      frame "Test DRV 26A" {
        w7129 = T11 {"command"="", "command data"=variant} ("element")
        w7122 = 26 ("DUT index(0-59)")
        w7155 = T11 {"command"="", "command data"=variant} ("element")
        n3237 = disable-structure shown="LOGGING==TRUE" {
          disable-tunnel: w7133 -> [w7170 _]
          frame condition #0 (active) {
            n3238 = Empty String/Path?(string/path=w7170) -> (empty?=w7173:bool)
            n3239 = Select(t="Quece timeout", s=w7173, f=w7170) -> (s? t:f=w7169:string)
            n3240 = call "string log (SubVI).vi"("Enum"=enum16{"Init", "Log", "Read"}."Log", "state Name"=w7169) -> ()  [unwired: 8 in, 2 out]
          }
          frame condition #1 {
          }
        }
        n3241 = Flush Queue(queue=w7134) -> (queue out=w7135:refnum<queue>)  [unwired: 1 in, 2 out]
        n3242 = Decrement(x=w7122) -> (x-1=w7126:i32)
        n3243 = Index Array(array=w7123, index=w7126) -> (element=w7124:refnum<vi>)
        n3244 = property class="ColBox"(reference=w7124, "Value"=u32 10000536 ("DRV 1")) -> ()  [unwired: 1 in, 2 out]
        n3245 = To Variant(anything=bool[] [FALSE, TRUE, FALSE, FALSE, FALSE, FALSE]) -> (Variant=w7152:variant)
        n3246 = To Variant(anything=T6."demux1_10_channel5" ("demux1_10(x6)_encode")) -> (Variant=w7156:variant)
        n3247 = To Variant(anything=T4."mux6_1_channel2_3" ("mux6_1(3wires)_encode")) -> (Variant=w7159:variant)
        n3248 = To Variant(anything=T5."mux10_1_channel5" ("mux10_1(x6)_encode")) -> (Variant=w7161:variant)
        n3249 = Bundle By Name(cluster=w7155, "command"="MEAS.mux10-1", "command data"=w7161) -> (w7150:T11)
        n3250 = Bundle By Name(cluster=w7155, "command"="MEAS.mux6_1", "command data"=w7159) -> (w7149:T11)
        n3251 = Bundle By Name(cluster=w7155, "command"="MEAS.demux1-10", "command data"=w7156) -> (w7148:T11)
        n3252 = Bundle By Name(cluster=w7155, "command"="MEAS.eMIC", "command data"=w7152) -> (w7147:T11)
        n3253 = Bundle By Name(cluster=w7155, "command"="MEAS.AllRelaysOFF") -> (w7151:T11)
        n3254 = Build Array(w7151, w7150, w7149, w7148, w7147) -> (w7142:T11[])
        n3255 = Bundle By Name(cluster=w7129, "command"="MEAS.requestAC", "command data"=w7122) -> (w7143:T11)
        n3256 = Bundle By Name(cluster=w7129, "command"="Apps.WaitForEvent", "command data"=w7122) -> (w7128:T11)
        n3257 = Bundle By Name(cluster=w7129, "command"="MEAS.DMM dual read") -> (w7144:T11)
        n3258 = Bundle By Name(cluster=w7129, "command"="Apps.UI Update 1") -> (w7130:T11)
        n3259 = Build Array(w7144, w7143, w7128, w7130) -> (w7141:T11[])
        n3260 = Build Array (concatenate)(w7142, w7141) -> (w7140:T11[])
        n3261 = for {
          tunnel: w7140 -> [w7177] mode=indexing
          tunnel: w7135 -> [w7178]
          tunnel: [w7174] -> w7138 mode=indexing
          n3262 = Unbundle By Name(w7177) -> ("command"=w7176:string, "command data"=w7175:variant)
          n3263 = call "App enquece.vi"("command data"=w7175, "command"=w7176, "queue in"=w7178) -> ("error out"=w7174:errorcluster)  [unwired: 7 in, 1 out]
        }
        n3264 = Merge Errors(w7139, w7138) -> (w7137:errorcluster)
      }
      frame "Test DRV 27A" {
        w7186 = T11 {"command"="", "command data"=variant} ("element")
        w7180 = 27 ("DUT index(0-59)")
        w7212 = T11 {"command"="", "command data"=variant} ("element")
        n3265 = disable-structure shown="LOGGING==TRUE" {
          disable-tunnel: w7190 -> [w7227 _]
          frame condition #0 (active) {
            n3266 = Empty String/Path?(string/path=w7227) -> (empty?=w7230:bool)
            n3267 = Select(t="Quece timeout", s=w7230, f=w7227) -> (s? t:f=w7226:string)
            n3268 = call "string log (SubVI).vi"("Enum"=enum16{"Init", "Log", "Read"}."Log", "state Name"=w7226) -> ()  [unwired: 8 in, 2 out]
          }
          frame condition #1 {
          }
        }
        n3269 = Flush Queue(queue=w7191) -> (queue out=w7192:refnum<queue>)  [unwired: 1 in, 2 out]
        n3270 = Decrement(x=w7180) -> (x-1=w7183:i32)
        n3271 = Index Array(array=w7179, index=w7183) -> (element=w7181:refnum<vi>)
        n3272 = property class="ColBox"(reference=w7181, "Value"=u32 10000536 ("DRV 1")) -> ()  [unwired: 1 in, 2 out]
        n3273 = To Variant(anything=bool[] [FALSE, FALSE, TRUE, FALSE, FALSE, FALSE]) -> (Variant=w7209:variant)
        n3274 = To Variant(anything=T6."demux1_10_channel5" ("demux1_10(x6)_encode")) -> (Variant=w7213:variant)
        n3275 = To Variant(anything=T4."mux6_1_channel3_3" ("mux6_1(3wires)_encode")) -> (Variant=w7216:variant)
        n3276 = To Variant(anything=T5."mux10_1_channel5" ("mux10_1(x6)_encode")) -> (Variant=w7218:variant)
        n3277 = Bundle By Name(cluster=w7212, "command"="MEAS.mux10-1", "command data"=w7218) -> (w7207:T11)
        n3278 = Bundle By Name(cluster=w7212, "command"="MEAS.mux6_1", "command data"=w7216) -> (w7206:T11)
        n3279 = Bundle By Name(cluster=w7212, "command"="MEAS.demux1-10", "command data"=w7213) -> (w7205:T11)
        n3280 = Bundle By Name(cluster=w7212, "command"="MEAS.eMIC", "command data"=w7209) -> (w7204:T11)
        n3281 = Bundle By Name(cluster=w7212, "command"="MEAS.AllRelaysOFF") -> (w7208:T11)
        n3282 = Build Array(w7208, w7207, w7206, w7205, w7204) -> (w7199:T11[])
        n3283 = Bundle By Name(cluster=w7186, "command"="MEAS.requestAC", "command data"=w7180) -> (w7200:T11)
        n3284 = Bundle By Name(cluster=w7186, "command"="Apps.WaitForEvent", "command data"=w7180) -> (w7185:T11)
        n3285 = Bundle By Name(cluster=w7186, "command"="MEAS.DMM dual read") -> (w7201:T11)
        n3286 = Bundle By Name(cluster=w7186, "command"="Apps.UI Update 1") -> (w7187:T11)
        n3287 = Build Array(w7201, w7200, w7185, w7187) -> (w7198:T11[])
        n3288 = Build Array (concatenate)(w7199, w7198) -> (w7197:T11[])
        n3289 = for {
          tunnel: w7197 -> [w7234] mode=indexing
          tunnel: w7192 -> [w7235]
          tunnel: [w7231] -> w7195 mode=indexing
          n3290 = Unbundle By Name(w7234) -> ("command"=w7233:string, "command data"=w7232:variant)
          n3291 = call "App enquece.vi"("command data"=w7232, "command"=w7233, "queue in"=w7235) -> ("error out"=w7231:errorcluster)  [unwired: 7 in, 1 out]
        }
        n3292 = Merge Errors(w7196, w7195) -> (w7194:errorcluster)
      }
      frame "Test DRV 28A" {
        w7243 = T11 {"command"="", "command data"=variant} ("element")
        w7236 = 28 ("DUT index(0-59)")
        w7269 = T11 {"command"="", "command data"=variant} ("element")
        n3293 = disable-structure shown="LOGGING==TRUE" {
          disable-tunnel: w7247 -> [w7284 _]
          frame condition #0 (active) {
            n3294 = Empty String/Path?(string/path=w7284) -> (empty?=w7287:bool)
            n3295 = Select(t="Quece timeout", s=w7287, f=w7284) -> (s? t:f=w7283:string)
            n3296 = call "string log (SubVI).vi"("Enum"=enum16{"Init", "Log", "Read"}."Log", "state Name"=w7283) -> ()  [unwired: 8 in, 2 out]
          }
          frame condition #1 {
          }
        }
        n3297 = Flush Queue(queue=w7248) -> (queue out=w7249:refnum<queue>)  [unwired: 1 in, 2 out]
        n3298 = Decrement(x=w7236) -> (x-1=w7240:i32)
        n3299 = Index Array(array=w7237, index=w7240) -> (element=w7238:refnum<vi>)
        n3300 = property class="ColBox"(reference=w7238, "Value"=u32 10000536 ("DRV 1")) -> ()  [unwired: 1 in, 2 out]
        n3301 = To Variant(anything=bool[] [FALSE, FALSE, FALSE, TRUE, FALSE, FALSE]) -> (Variant=w7266:variant)
        n3302 = To Variant(anything=T6."demux1_10_channel5" ("demux1_10(x6)_encode")) -> (Variant=w7270:variant)
        n3303 = To Variant(anything=T4."mux6_1_channel4_3" ("mux6_1(3wires)_encode")) -> (Variant=w7273:variant)
        n3304 = To Variant(anything=T5."mux10_1_channel5" ("mux10_1(x6)_encode")) -> (Variant=w7275:variant)
        n3305 = Bundle By Name(cluster=w7269, "command"="MEAS.mux10-1", "command data"=w7275) -> (w7264:T11)
        n3306 = Bundle By Name(cluster=w7269, "command"="MEAS.mux6_1", "command data"=w7273) -> (w7263:T11)
        n3307 = Bundle By Name(cluster=w7269, "command"="MEAS.demux1-10", "command data"=w7270) -> (w7262:T11)
